vi "PrintBuffer.vi"(6 "Number of Data Points":u32=10, 7 "SMU":T2, 8 "Error In":errorcluster, 9 "Buffer Value":T1, 10 "Buffer":u8=1 min=1 max=2 step=1, 11 "Kiethley 2602 In":refnum<visa-resource-name>) -> (0 "Error Out":errorcluster, 2 "Buffer":string, 3 "Keithley 2602 Out":refnum<visa-resource-name>)   [LabVIEW 2013, in "Keithley-2602.lvlib"]
uses:
  Keithley-2602.lvlib
  Controls/SMU.ctl
  Controls/BufferValue.ctl
panel:
  out "Command":string
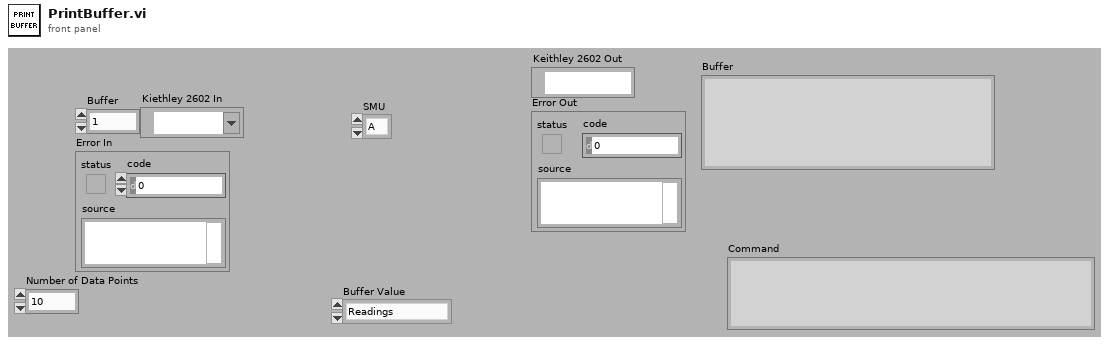
[diagram p1: front panel]
types:
  T1 = typedef "Keithley-2602.lvlib/BufferValue.ctl" = enum16{"Readings", "Source", "Timestamp"}
  T2 = typedef "Keithley-2602.lvlib/SMU.ctl" = enum16{"A", "B"}
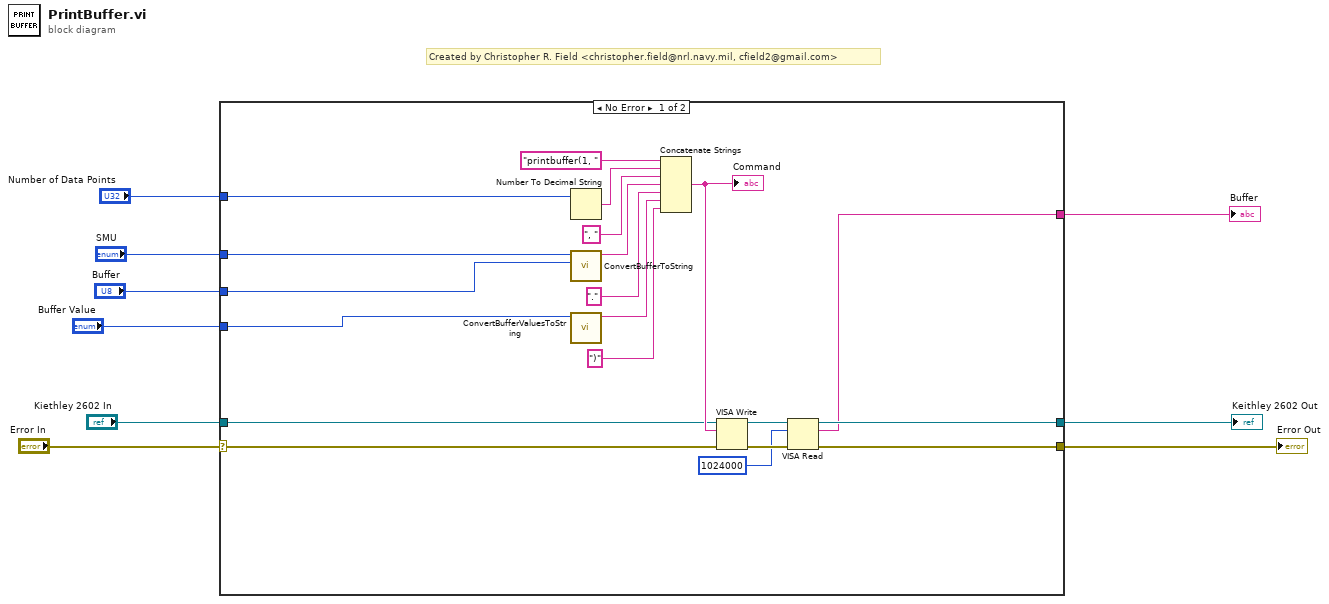
[diagram p0: block diagram]
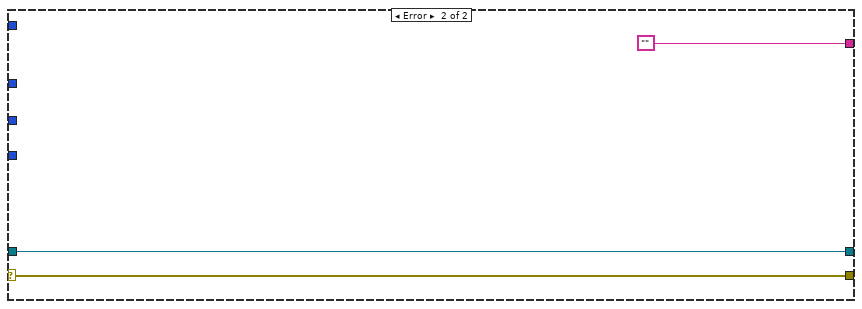
[diagram p2: hidden frame]
diagram:
  # "Created by Christopher R. Field <christopher.field@nrl.navy.mil, cfield2@gmail.com>"
  n1 = case shown="No Error" "Error In" {
    selector: "Error In" -> [w10 w30]
    tunnel: "Buffer" -> [w27 _]
    tunnel: [w20 w32] -> w8
    tunnel: [w19 w30] -> w7
    tunnel: [w18 ""] -> w6
    tunnel: "Kiethley 2602 In" -> [w14 w32]
    tunnel: "Number of Data Points" -> [w13 _]
    tunnel: "Buffer Value" -> [w12 _]
    tunnel: "SMU" -> [w11 _]
    frame No Error {
      n2 = Number To Decimal String(number=w13) -> (decimal integer string=w28:string)  [unwired: 1 in]
      n3 = call "ConvertBufferToString.vi"("Buffer"=w27, "SMU"=w11) -> ("Buffer"=w25:string)  [unwired: 9 in]
      n4 = call "ConvertBufferValuesToString.vi"("Buffer Value"=w12) -> ("Values"=w16:string)  [unwired: 10 in]
      n5 = Concatenate Strings("printbuffer(1, ", w28, ", " ("string"), w25, "." ("string"), w16, ")" ("string")) -> (w24:string)
      "Command" <- w24
      n6 = VISA Write(VISA resource name=w14, write buffer=w24, error in (no error)=w10) -> (VISA resource name out=w23:refnum<visa-resource-name>, error out=w22:errorcluster)  [unwired: 1 out]
      n7 = VISA Read(VISA resource name=w23, byte count=u32 1024000, error in (no error)=w22) -> (VISA resource name out=w20:refnum<visa-resource-name>, read buffer=w18:string, error out=w19:errorcluster)  [unwired: 1 out]
    }
    frame Error {
    }
  }
  "Keithley 2602 Out" <- w8
  "Error Out" <- w7
  "Buffer" <- w6
